vi "EnqueueMessage.vi"(7 "Priority? (F)":bool, 8 "error in (no error)":errorcluster, 9 "Data":variant, 10 "Message":string, 11 "queue in":T1) -> (0 "error out":errorcluster, 3 "queue out (copy)":T1)   [LabVIEW 2020]
uses:
  QueueRef.ctl
  Message.ctl
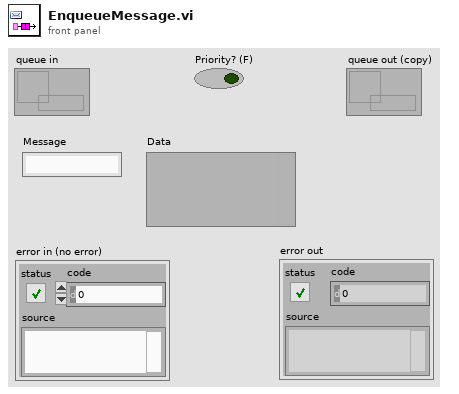
[diagram p1: front panel]
types:
  T1 = typedef "QueueRef.ctl" = refnum<queue>
  T2 = typedef "Message.ctl" = cluster{"Message":string, "data (variant)":variant}
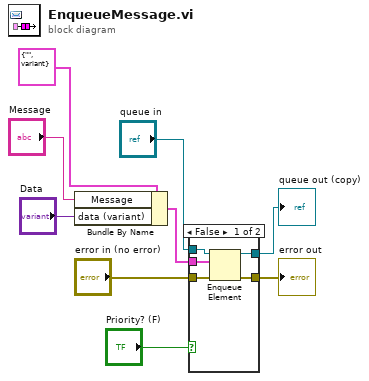
[diagram p0: block diagram]
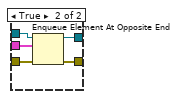
[diagram p2: hidden frame]
diagram:
  n1 = Bundle By Name(cluster=T2 {"Message"="", "data (variant)"=variant} ("Message Cluster"), "Message"="Message", "data (variant)"="Data") -> (w1:T2)
  n2 = case shown="False" "Priority? (F)" {
    tunnel: "queue in" -> [w14 w19]
    tunnel: [w13 w18] -> w7
    tunnel: "error in (no error)" -> [w12 w17]
    tunnel: [w11 w16] -> w5
    tunnel: w1 -> [w10 w15]
    frame False {
      n3 = Enqueue Element(queue=w14, element=w10, error in (no error)=w12) -> (queue out=w13:T1, error out=w11:errorcluster)  [unwired: 1 in, 1 out]
    }
    frame True {
      n4 = Enqueue Element At Opposite End(queue=w19, element=w15, error in (no error)=w17) -> (queue out=w18:T1, error out=w16:errorcluster)  [unwired: 1 in, 1 out]
    }
  }
  "queue out (copy)" <- w7
  "error out" <- w5
